vi "serialin.vi"() -> ()   [LabVIEW 2013]
uses:
  <vilib>/Instr/_visa.llb/VISA Configure Serial Port (Instr).vi
panel:
  out "Sensorausgaben":dbl[](graph)
  out "current sensor line":dbl[](array[numeric])
  out "current sensor line ASCII":string
  in  "sensor buffer":string
  out "element":string
  out "# elements in queue":i32
  in  "stop":bool
  in  "VISA resource name":refnum<visa-resource-name>
  in  "baud rate":u32=9600
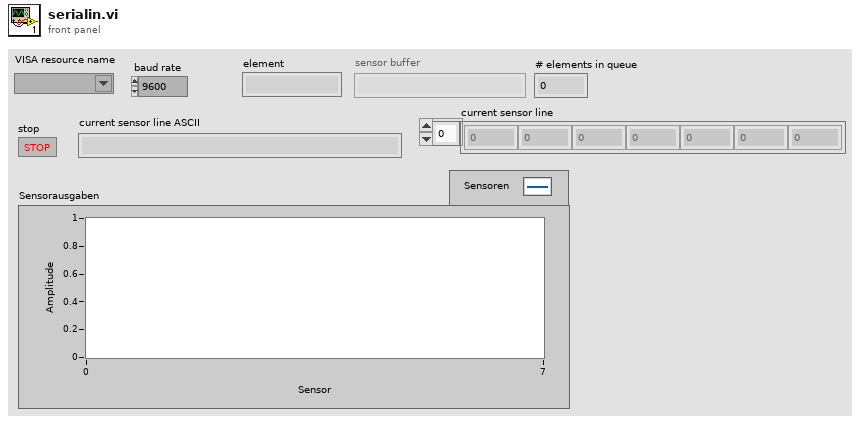
[diagram p1: front panel]
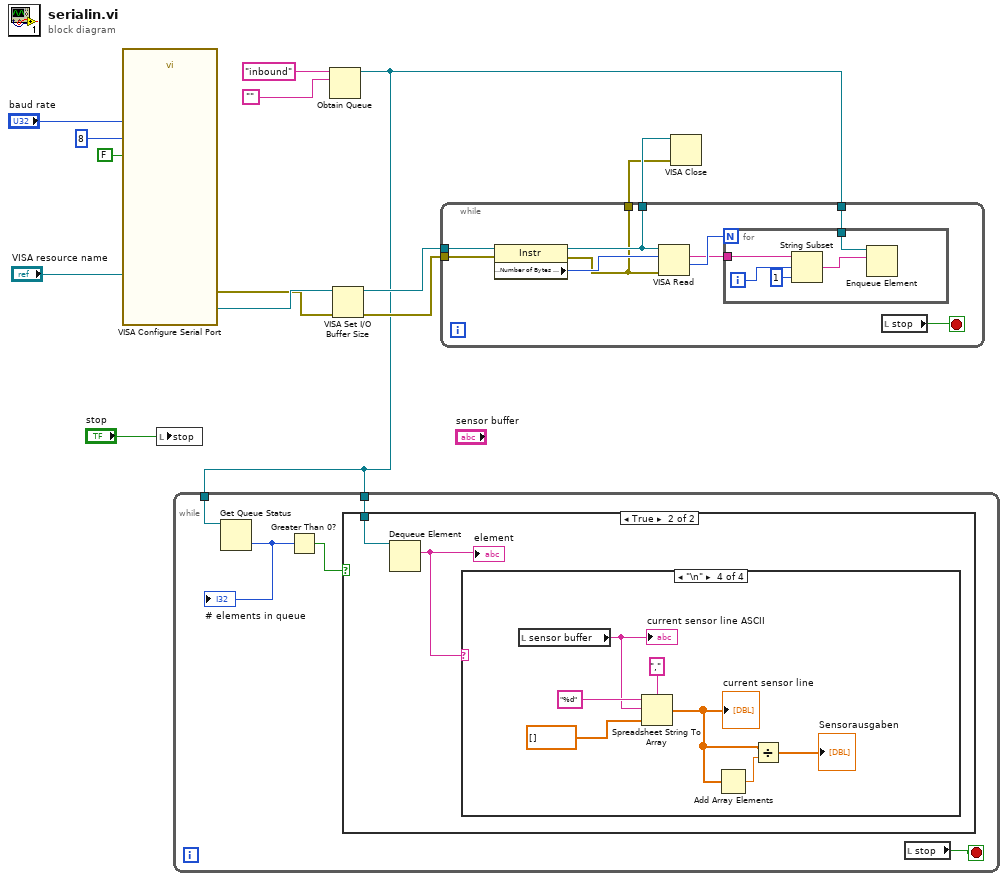
[diagram p0: block diagram]
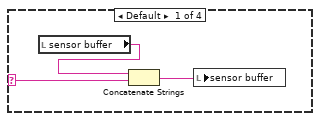
[diagram p3: hidden frame]
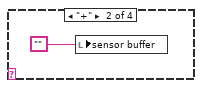
[diagram p4: hidden frame]
diagram:
  n1 = call-poly "VISA Configure Serial Port"("VISA resource name"="VISA resource name", "Enable Termination\nChar (T)"=FALSE ("Enable Termination\nChar (T)"), "baud rate (9600)"="baud rate", "data bits (8)"=u16 8) -> ("VISA resource name out"=w11:refnum<visa-resource-name>, "error out"=w10:errorcluster)  [unwired: 10 in]
  n2 = local write "stop"("stop") -> ()
  n3 = Obtain Queue(name (unnamed)="inbound", element data type="") -> (queue out=w1:refnum<queue>)  [unwired: 3 in, 2 out]
  n4 = while {
    tunnel: w1 -> [w18]
    tunnel: w1 -> [w15]
    stop <- w19 stop-if-true
    n5 = Get Queue Status(queue=w18) -> (# elements in queue=w17:i32)  [unwired: 2 in, 7 out]
    "# elements in queue" <- w17
    n6 = Greater Than 0?(x=w17) -> (x > 0?=w16:bool)
    n7 = case shown="True" w16 {
      tunnel: w15 -> [_ w21]
      frame False {
      }
      frame True {
        n8 = Dequeue Element(queue=w21) -> (element=w20:string)  [unwired: 2 in, 3 out]
        "element" <- w20
        n9 = case shown="\"\\n\"" w20 {
          selector: w20 -> [w22 _ _ _]
          frame Default {
            n10 = local read "sensor buffer"() -> (w23:string)
            n11 = Concatenate Strings(w23, w22) -> (w24:string)
            n12 = local write "sensor buffer"(w24) -> ()
          }
          frame "+" {
            n13 = local write "sensor buffer"("") -> ()
          }
          frame "\r" {
          }
          frame "\n" {
            n14 = local read "sensor buffer"() -> (w30:string)
            "current sensor line ASCII" <- w30
            n15 = Spreadsheet String To Array(delimiter (Tab)=",", format string="%d", spreadsheet string=w30, array type (2D Dbl)=dbl[] []) -> (array=w28:dbl[])
            "current sensor line" <- w28
            n16 = Add Array Elements(numeric array=w28) -> (sum=w27:dbl)
            n17 = Divide(x=w28, y=w27) -> (x/y=→"Sensorausgaben":dbl[])
          }
        }
      }
    }
    n18 = local read "stop"() -> (w19:bool)
  }
  n19 = VISA Set I/O Buffer Size(VISA resource name=w11, error in (no error)=w10) -> (VISA resource name out=w9:refnum<visa-resource-name>, error out=w8:errorcluster)  [unwired: 2 in]
  n20 = while {
    tunnel: w9 -> [w41]
    tunnel: w8 -> [w40]
    tunnel: [w38] -> w6
    tunnel: [w37] -> w5
    tunnel: w1 -> [w33]
    stop <- w36 stop-if-true
    n21 = property class="Instr"(reference=w41, error in=w40) -> (reference out=w38:refnum<visa-resource-name>, error out=w37:errorcluster, "Serial Settings:Number of Bytes at Serial Port"=w39:u32)
    n22 = VISA Read(VISA resource name=w38, byte count=w39, error in (no error)=w37) -> (read buffer=w34:string, return count=w35:u32)  [unwired: 2 out]
    n23 = for {
      N: w35 -> [_]
      tunnel: w34 -> [w46]
      tunnel: w33 -> [w43]
      i -> [w45]
      n24 = String Subset(string=w46, offset (0)=w45, length (rest)=1 ("length (rest)")) -> (substring=w42:string)
      n25 = Enqueue Element(queue=w43, element=w42) -> ()  [unwired: 2 in, 3 out]
    }
    n26 = local read "stop"() -> (w36:bool)
  }
  n27 = VISA Close(VISA resource name=w6, error in (no error)=w5) -> ()  [unwired: 1 out]
